vi "dfd_Convert MRate Params to String.vi"(5 "format string":string="%-+024.16e", 6 "width (-)":i16, 7 "indent order":i32, 11 "multirate filter in":T2={"mMRate_Structure"=enum."CIC", "mMRate_Mode"=0, "mMRate_Factor"=1, "mMRate_FIRParams"={"mMRate_FIR_H"=[], "mMRate_FIR_IsNyquist?"=FALSE, "mMRate_FIR_IsSymmetric?"=FALSE}, "mMRate_CICParams"={"mMRate_CIC_#Stage"=2, "mMRate_CIC_Lag"=1, "mMRate_CIC_Type"=enum."Lowpass"}, "mMRate_Order"=1, "mMRate_Version"="1.0", "mMRate_Comments"="1.0", "mMRate_RationalFactor"={"mMRate_L"=-1, "mMRate_M"=-1}, "mMRate_Fs"=0.0, "mMRate_Quantized?"=FALSE, "mMRate_QFilterGain"=1.0, "mMRate_CoefWl"=16, "mMRate_Scaling"={"mMRate_ScaleByPowerOf2?"=FALSE, "mMRate_ScaleType"=enum."Time Domain 1-Norm"}, "mMRate_InputWl"=0, "mMRate_OutputWl"=0, "mMRate_OutputMode"=enum."Nearest", "mMRate_MultMode"=enum."Truncated", "mMRate_BitPruning"=FALSE, "mMRate_GainWl"=16, "mMRate_OutputFwl"=0, "mMRate_SumIwl"=0, "mMRate_InputIwl "=16, "mMRate_SumWl"=32, "mMRate_CoefIwl"=0} {"mMRate_SumWl" min=1 max=32 step=1; "mMRate_InputIwl" min=1 max=32 step=1; "mMRate_GainWl" min=1 max=32 step=1; "mMRate_OutputWl" min=1 max=32 step=1; "mMRate_InputWl" min=1 max=32 step=1; "mMRate_CoefWl" min=1 max=32 step=1; "mMRate_Mode" items=["Default"=-1, "No Rate Change"=0, "Interpolation"=1, "Decimation"=2, "Interpolated"=3, "Rational"=4]}) -> (3 "string":string)   [LabVIEW 2017, in "NI_DigFilter_Process.lvlib"]
uses:
  <vilib>/addons/Digital Filter Design/NI_DigFilter_Process.lvlib
  <vilib>/addons/Digital Filter Design/_Objects.llb/DFD Multirate Filter Obj.ctl
  <vilib>/addons/Digital Filter Design/_Objects.llb/DFD Multirate Mode.ctl
  <vilib>/addons/Digital Filter Design/_Objects.llb/DFD Coef Norm Type.ctl
  <vilib>/addons/Digital Filter Design/_Objects.llb/DFD Round-off Mode.ctl
  <vilib>/addons/Digital Filter Design/_Objects.llb/DFD FXP MRate Multiply Mode.ctl
  <vilib>/addons/Digital Filter Design/_Objects.llb/DFD Multirate Filtering Mode.ctl
  <vilib>/addons/Digital Filter Design/NI_DigFilterLicensed.lvlib
panel:
  out "filtering mode":T1=2 items=["No Rate Change", "Interpolation", "Decimation"]
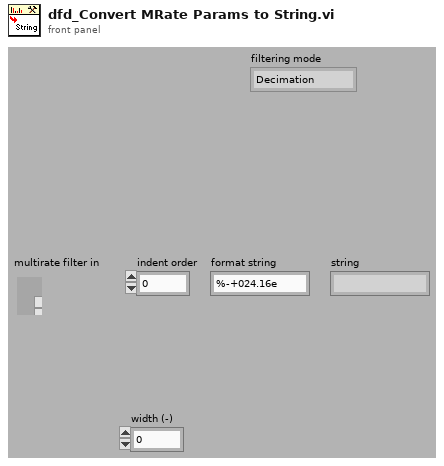
[diagram p1: front panel]
types:
  T1 = typedef "NI_DigFilterLicensed.lvlib/DFD Multirate Filtering Mode.ctl" = u16
  T2 = typedef "NI_DigFilterLicensed.lvlib/DFD Multirate Filter Obj.ctl" = cluster{"mMRate_Structure":enum16{"CIC", "FIR", "IIR", "Lattice"}, "mMRate_Mode":T3, "mMRate_Factor":i32, "mMRate_FIRParams":cluster{"mMRate_FIR_H":dbl[], "mMRate_FIR_IsNyquist?":bool, "mMRate_FIR_IsSymmetric?":bool}, "mMRate_CICParams":cluster{"mMRate_CIC_#Stage":i32, "mMRate_CIC_Lag":i32, "mMRate_CIC_Type":enum16{"Lowpass", "Highpass"}}, "mMRate_Order":i32, "mMRate_Version":string, "mMRate_Comments":string, "mMRate_RationalFactor":cluster{"mMRate_L":i32, "mMRate_M":i32}, "mMRate_Fs":dbl, "mMRate_Quantized?":bool, "mMRate_QFilterGain":dbl, "mMRate_CoefWl":i16, "mMRate_Scaling":cluster{"mMRate_ScaleByPowerOf2?":bool, "mMRate_ScaleType":T4}, "mMRate_InputWl":i16, "mMRate_OutputWl":i16, "mMRate_OutputMode":T5, "mMRate_MultMode":T6, "mMRate_BitPruning":bool, "mMRate_GainWl":i16, "mMRate_OutputFwl":i16, "mMRate_SumIwl":i16, "mMRate_InputIwl ":i16, "mMRate_SumWl":i16, "mMRate_CoefIwl":i16}
  T3 = typedef "NI_DigFilterLicensed.lvlib/DFD Multirate Mode.ctl" = i16
  T4 = typedef "NI_DigFilterLicensed.lvlib/DFD Coef Norm Type.ctl" = enum16{"No Norm", "Time Domain 1-Norm", "Time Domain 2-Norm", "Time Domain Inf-Norm"}
  T5 = typedef "NI_DigFilterLicensed.lvlib/DFD Round-off Mode.ctl" = enum16{"Nearest", "Truncation"}
  T6 = typedef "NI_DigFilterLicensed.lvlib/DFD FXP MRate Multiply Mode.ctl" = enum16{"Truncated", "Full"}
  T7 = cluster{"# stages":i32, "differential delay":i32, "filter type":enum16{"Lowpass", "Highpass"}}
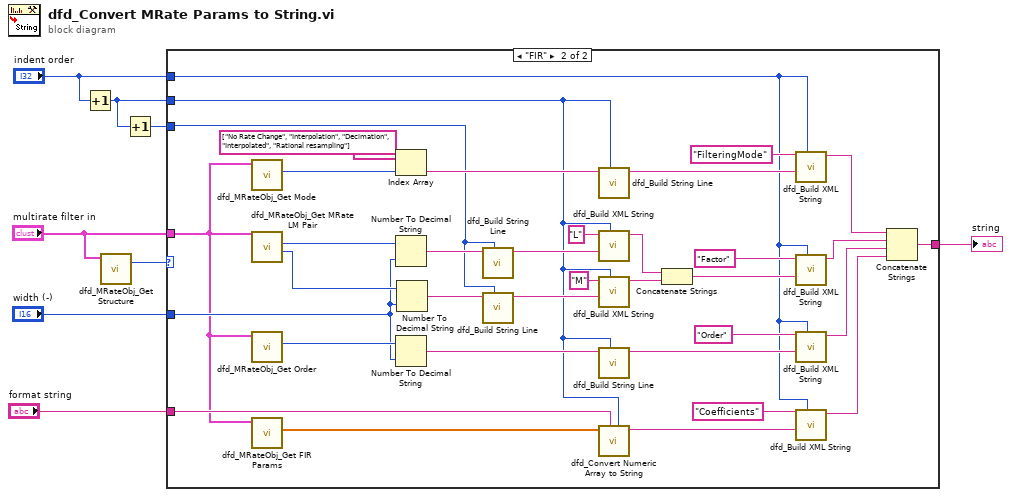
[diagram p0: block diagram]
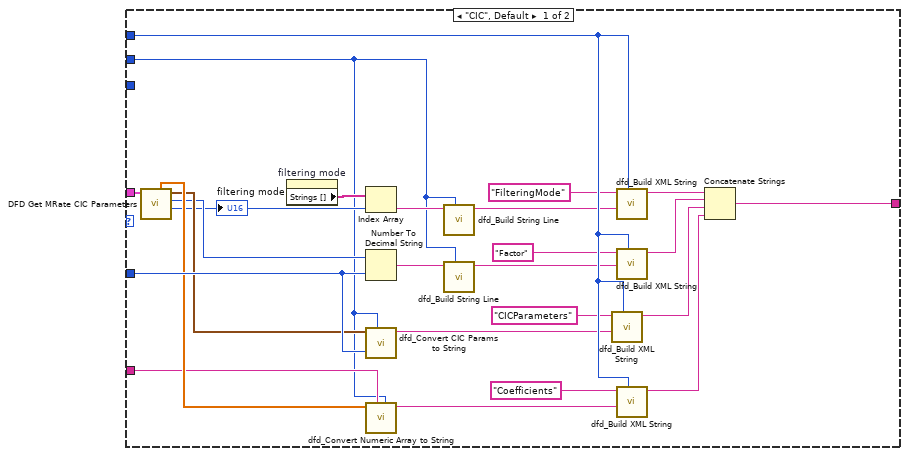
[diagram p2: hidden frame]
diagram:
  n1 = Increment(x="indent order") -> (x+1=w3:i32)
  n2 = call <vilib>:"dfd_MRateObj_Get Structure.vi"("multirate filter in"="multirate filter in") -> ("structure"=w6:enum16{"CIC", "FIR", "IIR", "Lattice"})  [unwired: 10 out]
  n3 = Increment(x=w3) -> (x+1=w2:i32)
  n4 = case shown="\"FIR\"" w6 {
    tunnel: "multirate filter in" -> [w33 w35]
    tunnel: "width (-)" -> [w32 w42]
    tunnel: "indent order" -> [w31 w45]
    tunnel: [w30 w49] -> w7
    tunnel: w3 -> [w11 w36]
    tunnel: "format string" -> [w12 w41]
    tunnel: w2 -> [_ w40]
    frame "CIC", Default {
      n5 = call <vilib>:"DFD Get MRate CIC Parameters.vi"("multirate filter in"=w33) -> ("filtering mode"=w23:T1, "factor"=w25:i32, "CIC parameters"=w27:T7, "h(n)"=w29:dbl[])  [unwired: 1 in, 6 out]
      "filtering mode" <- w23
      n6 = property on="filtering mode" class="Ring (strict)"() -> ("Strings []"=w24:string[])  [unwired: 2 in, 2 out]
      n7 = Index Array(array=w24, index=w23) -> (element=w21:string)
      n8 = Number To Decimal String(number=w25, width (-)=w32) -> (decimal integer string=w22:string)
      n9 = call <vilib>:"dfd_Convert CIC Params to String.vi"("width (-)"=w32, "indent order"=w11, "CIC params"=w27) -> ("string"=w9:string)  [unwired: 8 out]
      n10 = call <vilib>:"dfd_Convert Numeric Array to String.vi"("indent order"=w11, "format string"=w12, "numeric array"=w29) -> ("string"=w10:string)  [unwired: 1 in, 7 out]
      n11 = call <vilib>:"dfd_Build String Line.vi"("indent order"=w11, "string"=w21) -> ("string line"=w19:string)  [unwired: 9 out]
      n12 = call <vilib>:"dfd_Build String Line.vi"("indent order"=w11, "string"=w22) -> ("string line"=w20:string)  [unwired: 9 out]
      n13 = call <vilib>:"dfd_Build XML String.vi"("indent order"=w31, "string in"=w9, "element name"="CICParameters") -> ("xml string out"=w13:string)  [unwired: 2 in, 6 out]
      n14 = call <vilib>:"dfd_Build XML String.vi"("indent order"=w31, "string in"=w19, "element name"="FilteringMode") -> ("xml string out"=w15:string)  [unwired: 2 in, 6 out]
      n15 = call <vilib>:"dfd_Build XML String.vi"("indent order"=w31, "string in"=w20, "element name"="Factor") -> ("xml string out"=w14:string)  [unwired: 2 in, 6 out]
      n16 = call <vilib>:"dfd_Build XML String.vi"("indent order"=w31, "string in"=w10, "element name"="Coefficients") -> ("xml string out"=w16:string)  [unwired: 2 in, 6 out]
      n17 = Concatenate Strings(w15, w14, w13, w16) -> (w30:string)
    }
    frame "FIR" {
      n18 = call <vilib>:"dfd_MRateObj_Get Mode.vi"("multirate filter in"=w35) -> ("mode"=w68:T3)  [unwired: 10 out]
      n19 = call <vilib>:"dfd_MRateObj_Get MRate LM Pair.vi"("multirate filter in"=w35) -> ("M"=w63:i32, "L"=w64:i32)  [unwired: 1 in, 8 out]
      n20 = call <vilib>:"dfd_MRateObj_Get Order.vi"("multirate filter in"=w35) -> ("order"=w54:i32)  [unwired: 10 out]
      n21 = call <vilib>:"dfd_MRateObj_Get FIR Params.vi"("multirate filter in"=w35) -> ("h(n)"=w38:dbl[])  [unwired: 10 out]
      n22 = Index Array(array=string[] ["No Rate Change", "Interpolation", "Decimation", "Interpolated", "Rational resampling"] ("Strings []"), index=w68) -> (element=w67:string)
      n23 = Number To Decimal String(number=w64, width (-)=w42) -> (decimal integer string=w62:string)
      n24 = Number To Decimal String(number=w54, width (-)=w42) -> (decimal integer string=w53:string)
      n25 = Number To Decimal String(number=w63, width (-)=w42) -> (decimal integer string=w61:string)
      n26 = call <vilib>:"dfd_Build String Line.vi"("indent order"=w40, "string"=w62) -> ("string line"=w59:string)  [unwired: 9 out]
      n27 = call <vilib>:"dfd_Build String Line.vi"("indent order"=w40, "string"=w61) -> ("string line"=w60:string)  [unwired: 9 out]
      n28 = call <vilib>:"dfd_Build String Line.vi"("indent order"=w36, "string"=w67) -> ("string line"=w66:string)  [unwired: 9 out]
      n29 = call <vilib>:"dfd_Build XML String.vi"("indent order"=w36, "string in"=w59, "element name"="L") -> ("xml string out"=w58:string)  [unwired: 2 in, 6 out]
      n30 = call <vilib>:"dfd_Build XML String.vi"("indent order"=w36, "string in"=w60, "element name"="M") -> ("xml string out"=w57:string)  [unwired: 2 in, 6 out]
      n31 = call <vilib>:"dfd_Build String Line.vi"("indent order"=w36, "string"=w53) -> ("string line"=w52:string)  [unwired: 9 out]
      n32 = call <vilib>:"dfd_Convert Numeric Array to String.vi"("indent order"=w36, "format string"=w41, "numeric array"=w38) -> ("string"=w37:string)  [unwired: 3 in, 5 out]
      n33 = Concatenate Strings(w58, w57) -> (w56:string)
      n34 = call <vilib>:"dfd_Build XML String.vi"("indent order"=w45, "string in"=w66, "element name"="FilteringMode") -> ("xml string out"=w50:string)  [unwired: 2 in, 6 out]
      n35 = call <vilib>:"dfd_Build XML String.vi"("indent order"=w45, "string in"=w56, "element name"="Factor") -> ("xml string out"=w48:string)  [unwired: 2 in, 6 out]
      n36 = call <vilib>:"dfd_Build XML String.vi"("indent order"=w45, "string in"=w52, "element name"="Order") -> ("xml string out"=w47:string)  [unwired: 2 in, 6 out]
      n37 = call <vilib>:"dfd_Build XML String.vi"("indent order"=w45, "string in"=w37, "element name"="Coefficients") -> ("xml string out"=w46:string)  [unwired: 2 in, 6 out]
      n38 = Concatenate Strings(w50, w48, w47, w46) -> (w49:string)
    }
  }
  "string" <- w7
